vi "Expt-2.vi"() -> ()   [LabVIEW 2020]
panel:
  out "current time":timestamp
  out "x = 0?":bool
  in  "Numeric 2":dbl
  in  "Numeric 1":dbl
  out "x > y?":bool
  in  "y":dbl
  in  "x":dbl
  out "result 2":bool
  in  "Boolean 6":bool
  in  "Boolean 5":bool
  in  "Boolean 4":bool
  out "result":bool
  in  "Boolean 3":bool
  in  "Boolean 2":bool
  in  "Boolean":bool
  # "AND GATE"
  # "OR GATE"
  # "1)"
  # "2)"
  # "3)"
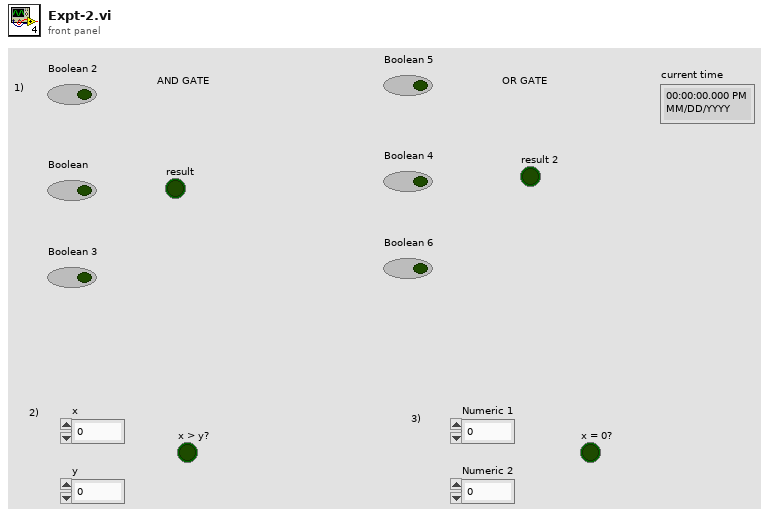
[diagram p1: front panel]
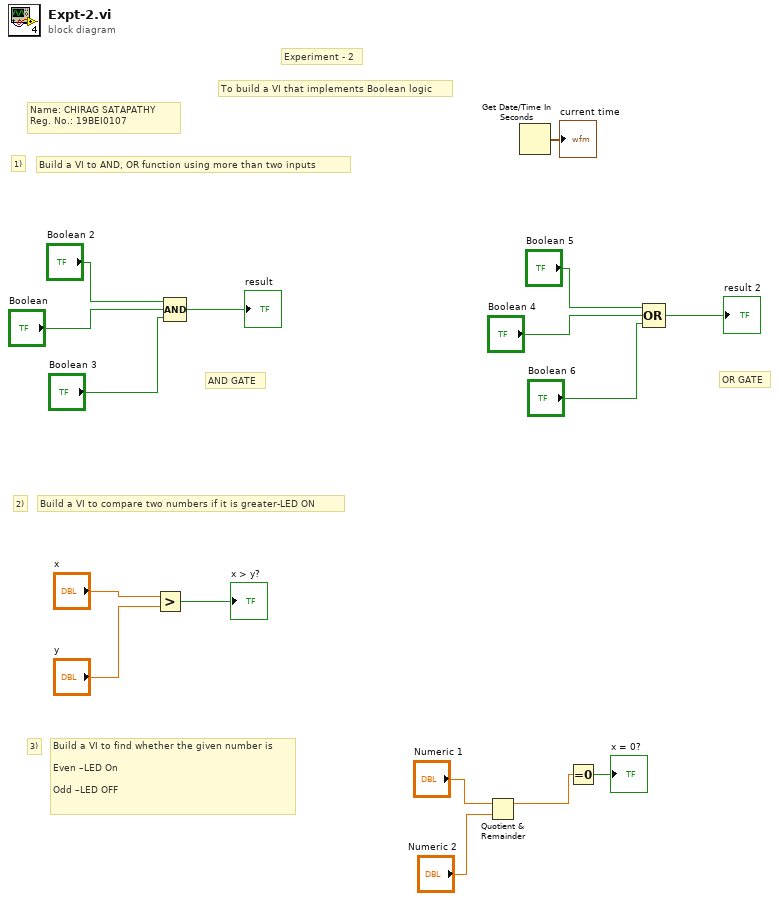
[diagram p0: block diagram]
diagram:
  # "Name: CHIRAG SATAPATHY\nReg. No.: 19BEI0107"
  # "Build a VI to find whether the given number is\n\nEven –LED On\n\nOdd –LED OFF"
  # "3)"
  # "Build a VI to compare two numbers if it is greater-LED ON"
  # "2)"
  # "OR GATE"
  # "AND GATE"
  # "Build a VI to AND, OR function using more than two inputs"
  # "1)"
  # "Experiment - 2"
  # "To build a VI that implements Boolean logic"
  n1 = Greater?(x="x", y="y") -> (0:→"x > y?":bool)
  n2 = Compound Arithmetic op=AND("Boolean 2", "Boolean", "Boolean 3") -> (→"result":bool)
  n3 = Quotient & Remainder(x="Numeric 1", y="Numeric 2") -> (x-y*floor(x/y)=w2:dbl)  [unwired: 1 out]
  n4 = Get Date/Time In Seconds() -> (seconds since 1Jan1904=→"current time":timestamp)
  n5 = Equal To 0?(x=w2) -> (x = 0?=→"x = 0?":bool)
  n6 = Compound Arithmetic op=OR("Boolean 5", "Boolean 4", "Boolean 6") -> (→"result 2":bool)
